vi "STM Comm Close All Connections.vi"(7 "Name":string, 8 "error in":errorcluster, 10 "TCP Ref":T1, 11 "listener ID":refnum<k5>) -> (0 "error out":errorcluster)   [LabVIEW 2015, in "Control Addon Engine.lvlib" / "STM.lvlib"]
uses:
  STM.lvlib
  STM Comm Lookup Table_Ref.ctl
  <userlib>/STM/Connection Manager/TCP/stm_TCPConnectionMethod.ctl
  <vilib>/NI Veristand/Custom Device Tools/Custom Device Utility Library/Custom Device Utility Library.lvlib
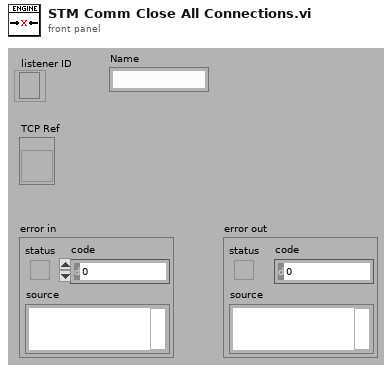
[diagram p1: front panel]
types:
  T1 = typedef "Control Addon Engine.lvlib/STM.lvlib/STM Comm Lookup Table_Ref.ctl" = refnum<vi>
  T2 = typedef "stm_TCPConnectionMethod.ctl" = enum16{"Initialize", "Add Connection", "Set Properties", "Get Connection(s)", "Remove Connection", "Remove All Connections", "Get Connection Count"}
  T3 = typedef "stm_TCP Connection Info.ctl" = cluster{"connection ID":refnum<k5>, "Meta data":T4[]}
  T4 = typedef "stm_MetaDataElement.ctl" = string
  T5 = typedef "stm_TCPConnectionProperties.ctl" = cluster{"Name":string, "Address":string, "Custom":string}
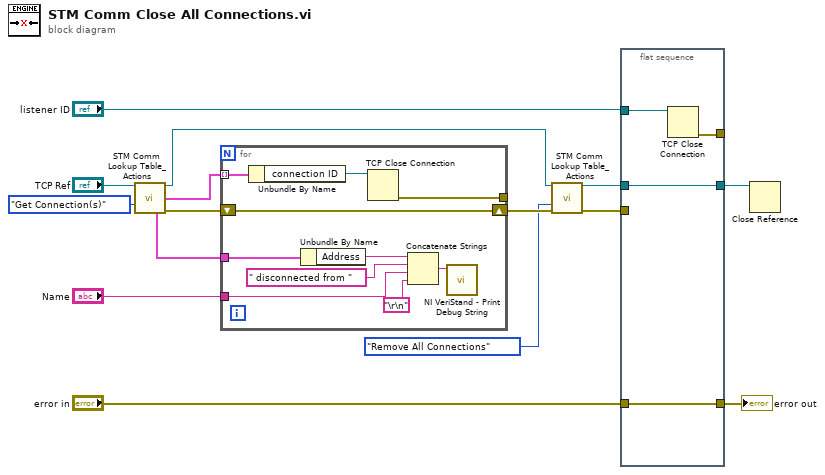
[diagram p0: block diagram]
diagram:
  n1 = call "STM Comm Lookup Table_Actions.vi"("vi reference"="TCP Ref", "Method"=stm_TCPConnectionMethod."Get Connection(s)") -> ("vi reference"=w5:T1, "All Connections"=w12:T3[], "Properties out"=w3:T5, "error out"=w11:errorcluster)  [unwired: 7 in, 3 out]
  n2 = for {
    tunnel: w12 -> [w17] mode=indexing
    shift-right: [w23] -> w10
    shift-left: w11 -> [w23]
    tunnel: [w24] -> _
    tunnel: "Name" -> [w19]
    tunnel: w3 -> [w18]
    n3 = Unbundle By Name(w17) -> ("connection ID"=w25:refnum<k5>)
    n4 = Unbundle By Name(w18) -> ("Address"=w20:string)
    n5 = TCP Close Connection(connection ID=w25) -> (error out=w24:errorcluster)  [unwired: 2 in, 1 out]
    n6 = Concatenate Strings(w20, " disconnected from " ("string"), w19, "\r\n") -> (w22:string)
    n7 = call <vilib>:"NI VeriStand - Print Debug String.vi"("Message"=w22) -> ()  [unwired: 10 in, 1 out]
  }
  n8 = call "STM Comm Lookup Table_Actions.vi"("vi reference"=w5, "Method"=stm_TCPConnectionMethod."Remove All Connections", "error in (no error)"=w10) -> ("vi reference"=w7:T1, "error out"=w9:errorcluster)  [unwired: 6 in, 5 out]
  n9 = flat-sequence {
    tunnel: "listener ID" -> [w29]
    tunnel: [w28] -> w14
    tunnel: w9 -> [_]
    tunnel: "error in" -> [w28]
    tunnel: [w27] -> _
    tunnel: w7 -> [w26]
    tunnel: [w26] -> w6
    frame #0 {
      n10 = TCP Close Connection(connection ID=w29) -> (error out=w27:errorcluster)  [unwired: 2 in, 1 out]
    }
  }
  n11 = Close Reference(reference=w6) -> ()  [unwired: 1 in, 1 out]
  "error out" <- w14
